vi "close.vi"(8 "error in (no error)":errorcluster, 11 "Generic Handler in":refnum<class "Generic Handler.lvclass">) -> (0 "error out":errorcluster, 3 "Generic Handler out":refnum<class "Generic Handler.lvclass">)   [LabVIEW 2025, in "Generic Handler.lvclass"]
uses:
  Generic Handler.lvclass
  Generic Handler.lvclass/Generic Handler.ctl
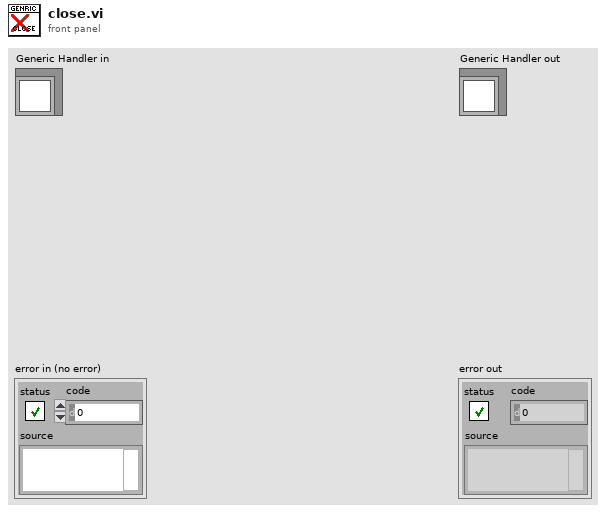
[diagram p1: front panel]
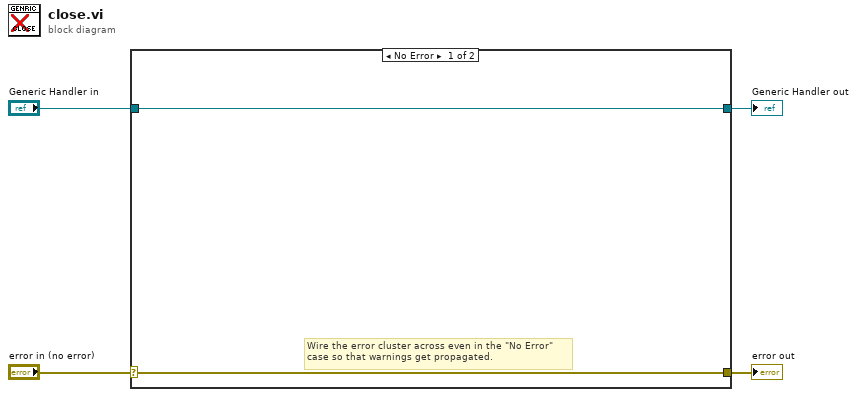
[diagram p0: block diagram]
diagram:
  n1 = case shown="No Error" "error in (no error)" {
    selector: "error in (no error)" -> [w5 w8]
    tunnel: [w5 w8] -> w3
    tunnel: [w6 w7] -> w1
    tunnel: "Generic Handler in" -> [w6 w7]
    frame No Error {
      # "Wire the error cluster across even in the \"No Error\"\ncase so that warnings get propagated."
    }
    frame Error {
    }
  }
  "error out" <- w3
  "Generic Handler out" <- w1
